vi "To Float Tree Data.vi"(10 "Float":dbl) -> (3 "Float Tree Data":refnum<class "Float.lvclass">)   [LabVIEW 2016, in "Float.lvclass"]
uses:
  Float.lvclass
  Float.lvclass/Float.ctl
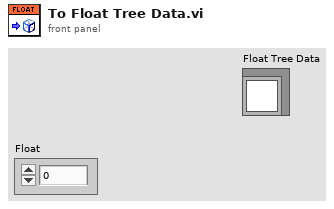
[diagram p1: front panel]
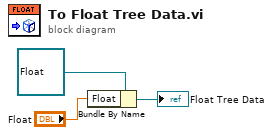
[diagram p0: block diagram]
diagram:
  n1 = Bundle By Name(cluster=refnum<class "Float.lvclass"> refnum ("Float in"), "Float"="Float") -> (→"Float Tree Data":refnum<class "Float.lvclass">)
